vi "Get Error Handler.vi"(8 "error in (no error)":errorcluster, 11 "Process In":refnum<class "Process.lvclass">) -> (0 "error out":errorcluster, 2 "Error Handler":refnum<class "Error Handler Interface.lvclass">, 3 "Process Out":refnum<class "Process.lvclass">)   [LabVIEW 2020, in "Process.lvclass"]
doc: "Returns the error handler configured for the process using the Set Error Handler.vi method."
uses:
  Process.lvclass
  Error Handler Interface/Error Handler Interface.lvclass
  Process.lvclass/Process.ctl
  <vilib>/Utility/error.llb/Clear Errors.vi
  Private/SubVIs/Enqueue Request Message.vi
  <vilib>/Utility/error.llb/Error Cluster From Error Code.vi
  Private/SubVIs/Wait for Response Message.vi
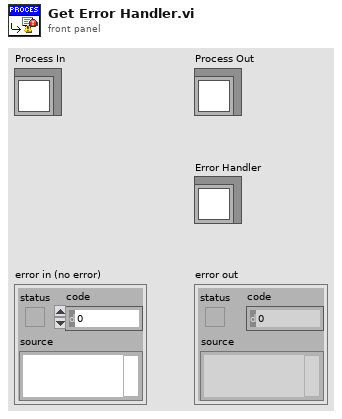
[diagram p1: front panel]
types:
  T1 = typedef "Process.lvclass/Lifecycle State.ctl" = enum16{"Uninitialized", "Initialized", "Started", "Running", "Stopped", "Finished"}
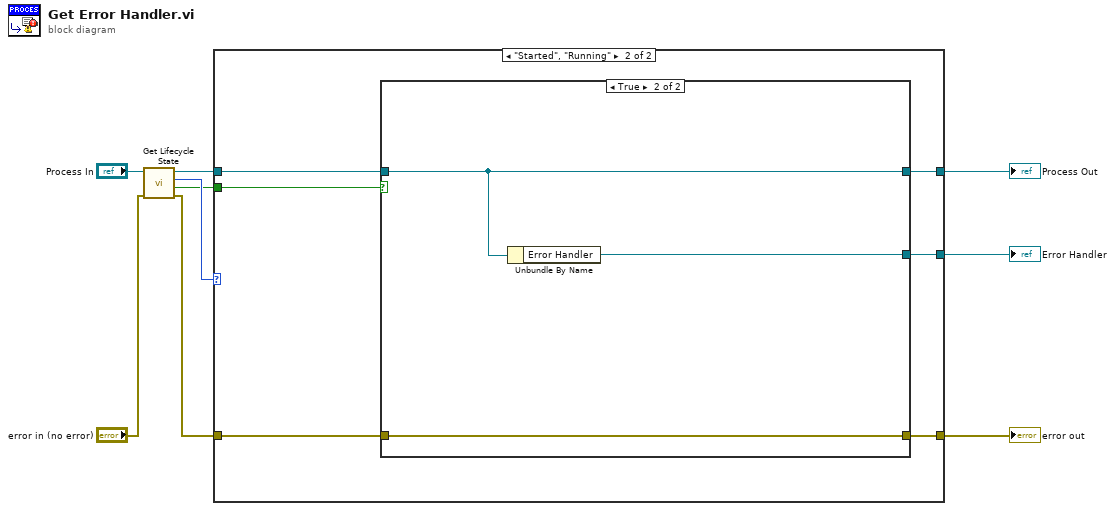
[diagram p0: block diagram]
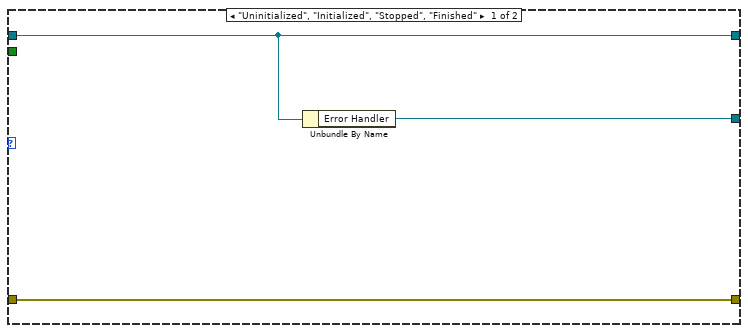
[diagram p2: hidden frame]
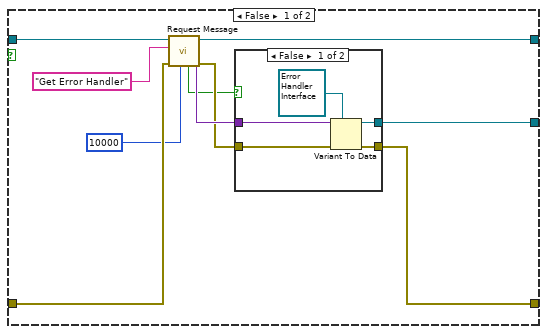
[diagram p3: hidden frame]
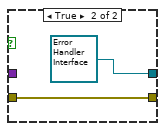
[diagram p4: hidden frame]
diagram:
  n1 = call "Get Lifecycle State.vi"("error in (no error)"="error in (no error)", "Process In"="Process In") -> ("error out"=w2:errorcluster, "In Process Loop?"=w1:bool, "Lifecycle State"=w4:T1, "Process Out"=w5:refnum<class "Process.lvclass">)  [unwired: 6 in]
  n2 = case shown="\"Started\", \"Running\"" w4 {
    tunnel: [w12 w18] -> w8
    tunnel: w2 -> [w10 w17]
    tunnel: [w11 w16] -> w7
    tunnel: [w10 w15] -> w6
    tunnel: w5 -> [w12 w14]
    tunnel: w1 -> [_ w13]
    frame "Uninitialized", "Initialized", "Stopped", "Finished" {
      n3 = Unbundle By Name(w12) -> ("Error Handler"=w11:refnum<class "Error Handler Interface.lvclass">)
    }
    frame "Started", "Running" {
      n4 = case shown="True" w13 {
        tunnel: [w28 w38] -> w18
        tunnel: w17 -> [w26 w36]
        tunnel: [w25 w37] -> w16
        tunnel: [w22 w36] -> w15
        tunnel: w14 -> [w20 w38]
        frame False {
          n5 = call "Request Message.vi"("timeout in ms (-1)"=10000, "error in (no error)"=w26, "Request Message"="Get Error Handler", "Process In"=w20) -> ("error out"=w23:errorcluster, "Response Message Data"=w24:variant, "Process Out"=w28:refnum<class "Process.lvclass">, "Timed out?"=w19:bool)  [unwired: 3 in, 1 out]
          n6 = case shown="False" w19 {
            tunnel: [w32 refnum<class "Error Handler Interface.lvclass"> refnum ("Error Handler")] -> w25
            tunnel: w24 -> [w31 _]
            tunnel: w23 -> [w30 w35]
            tunnel: [w29 w35] -> w22
            frame False {
              n7 = Variant To Data(error in=w30, type=refnum<class "Error Handler Interface.lvclass"> refnum ("Error Handler"), Variant=w31) -> (data=w32:refnum<class "Error Handler Interface.lvclass">, error out=w29:errorcluster)
            }
            frame True {
            }
          }
        }
        frame True {
          n8 = Unbundle By Name(w38) -> ("Error Handler"=w37:refnum<class "Error Handler Interface.lvclass">)
        }
      }
    }
  }
  "error out" <- w6
  "Process Out" <- w8
  "Error Handler" <- w7
